vi "Shutdown.vi"(8 "error in (no error)":errorcluster, 11 "DemoStage in":refnum<class "DemoStage.lvclass">) -> (0 "error out":errorcluster, 3 "DemoStage out":refnum<class "DemoStage.lvclass">)   [LabVIEW 2020, in "DemoStage.lvlib" / "DemoStage.lvclass"]
uses:
  DemoStage.lvclass
  Hardware Abstraction Layer/Component/Stage/Stage/Stage.lvclass
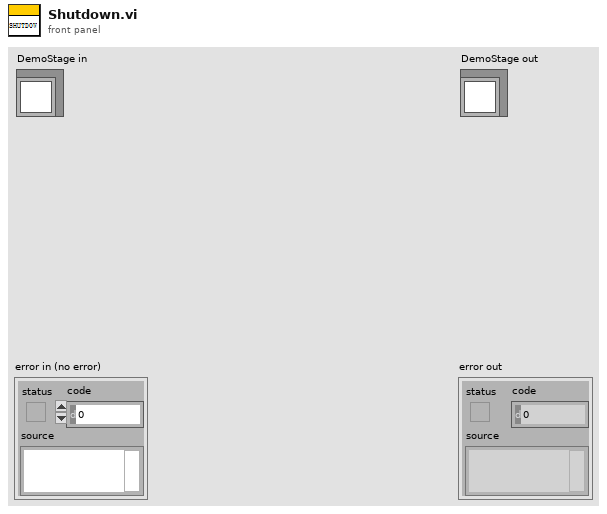
[diagram p1: front panel]
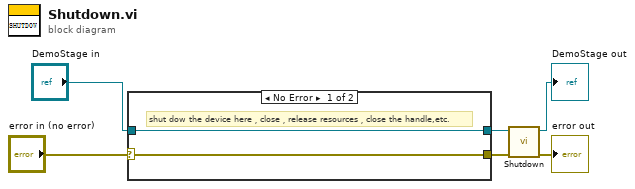
[diagram p0: block diagram]
diagram:
  n1 = case shown="No Error" "error in (no error)" {
    selector: "error in (no error)" -> [w7 w10]
    tunnel: [w7 w10] -> w3
    tunnel: [w8 w9] -> w4
    tunnel: "DemoStage in" -> [w8 w9]
    frame No Error {
      # "shut dow the device here，close，release resources，close the handle,etc."
    }
    frame Error {
    }
  }
  n2 = call-parent "Shutdown.vi"("error in (no error)"=w3, "Device in"=w4) -> ("error out"=→"error out":errorcluster, "Device out"=→"DemoStage out":refnum<class "DemoStage.lvclass">)  [unwired: 8 in]
